vi "Example_DAQ.vi"() -> ()   [LabVIEW 2021]
uses:
  DAQ_Control_1.ctl
  DAQ_Control_2.ctl
  DAQ_Control_3 .ctl
panel:
  in  "Time Unit":T1={"Time Unit"=enum."MicroSecond"}
  in  "Sampling data":T2={"Sample Numbers"=20000000, "Sample  Frequency (Hz)"=10000000}
  in  "Filename (ini)":string="Config_Ver_1\\pulse_sequence_DAQ.ini"
  out "Period (s )":dbl=2.0
  in  "Error  in":errorcluster
  out "Final Sending Data":u32[](array[numeric])
  out "error out":errorcluster
  in  "Digital Ports":tag="Dev1/port0"
  out "Sample Frequency (Hz)":u32=10000000 max=20000000 step=1
  out "Sample Numbers":u32=20000001
  in  "Sequence":T3
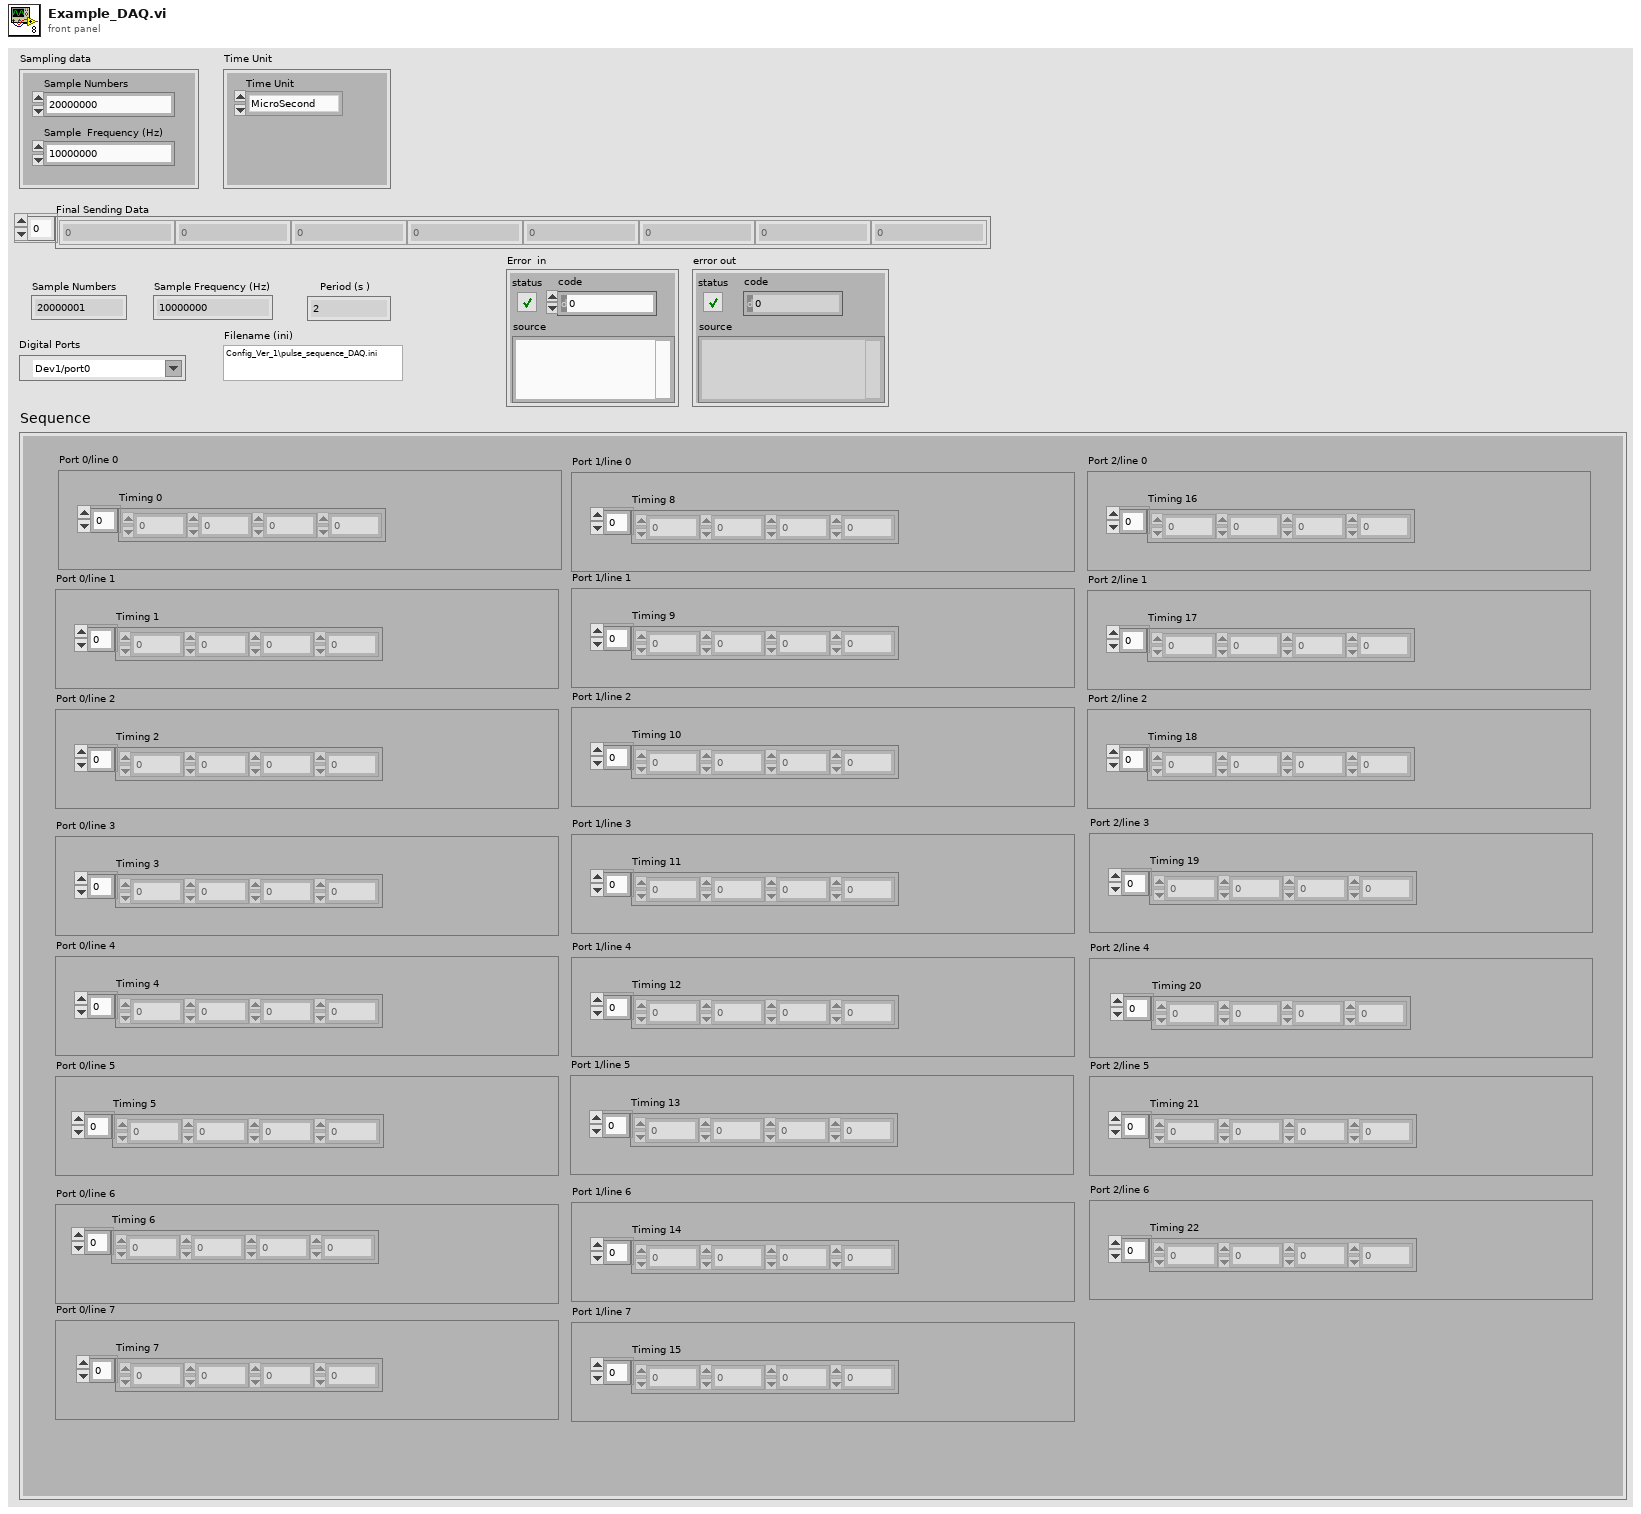
[diagram p1: front panel]
types:
  T1 = typedef "DAQ_Control_3 .ctl" = cluster{"Time Unit":enum16{"NanoSecond", "MicroSecond", "MilliSecond"}}
  T2 = typedef "DAQ_Control_2.ctl" = cluster{"Sample Numbers":u32, "Sample  Frequency (Hz)":u32}
  T3 = typedef "DAQ_Control_1.ctl" = cluster{"Port 2/line 6":cluster{"Timing 22":dbl[]}, "Port 2/line 5":cluster{"Timing 21":dbl[]}, "Port 2/line 4":cluster{"Timing 20":dbl[]}, "Port 2/line 3":cluster{"Timing 19":dbl[]}, "Port 2/line 2":cluster{"Timing 18":dbl[]}, "Port 2/line 1":cluster{"Timing 17":dbl[]}, "Port 2/line 0":cluster{"Timing 16":dbl[]}, "Port 1/line 7":cluster{"Timing 15":dbl[]}, "Port 1/line 6":cluster{"Timing 14":dbl[]}, "Port 1/line 5":cluster{"Timing 13":dbl[]}, "Port 1/line 4":cluster{"Timing 12":dbl[]}, "Port 1/line 3":cluster{"Timing 11":dbl[]}, "Port 1/line 2":cluster{"Timing 10":dbl[]}, "Port 1/line 1":cluster{"Timing 9":dbl[]}, "Port 1/line 0":cluster{"Timing 8":dbl[]}, "Port 0/line 7":cluster{"Timing 7\n":dbl[]}, "Port 0/line 6":cluster{"Timing 6\n":dbl[]}, "Port 0/line 5":cluster{"Timing 5\n":dbl[]}, "Port 0/line 4":cluster{"Timing 4\n":dbl[]}, "Port 0/line 3":cluster{"Timing 3\n":dbl[]}, "Port 0/line 2":cluster{"Timing 2":dbl[]}, "Port 0/line 1":cluster{"Timing 1\n":dbl[]}, "Port 0/line 0":cluster{"Timing 0":dbl[]}}
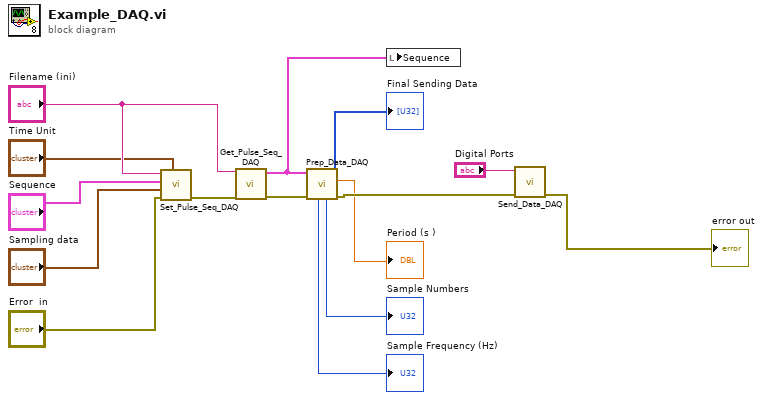
[diagram p0: block diagram]
diagram:
  n1 = call "Set_Pulse_Seq_DAQ.vi"("Time Unit"="Time Unit", "error in"="Error  in", "Sampling data"="Sampling data", "Sequence"="Sequence", "Filename (ini)"="Filename (ini)") -> ("error out"=w2:errorcluster)  [unwired: 6 in]
  n2 = call "Get_Pulse_Seq_DAQ.vi"("error in"=w2, "Filename (ini)"="Filename (ini)") -> ("error out"=w8:errorcluster, "data"=w4:T3)  [unwired: 8 in]
  n3 = call "Prep_Data_DAQ.vi"("Error  in"=w8, "Sequence"=w4) -> ("Error out"=w13:errorcluster, "Period (s )=Sample Numbers / Sample Frequency"=→"Period (s )":dbl, "Final Sending Data"=→"Final Sending Data":u32[], "Sample Numbers"=→"Sample Numbers":u32, "Sample Frequency (Hz)"=→"Sample Frequency (Hz)":u32)  [unwired: 4 in, 1 out]
  n4 = local write "Sequence"(w4) -> ()
  n5 = call "Send_Data_DAQ.vi"("error in"=w13, "Digital Ports"="Digital Ports") -> ("error out"=→"error out":errorcluster)  [unwired: 8 in, 1 out]
